vi "iWorx - Water Quality Lab.vi"() -> ()   [LabVIEW 2012]
uses:
  vi.lib/iWorx/iWorx Set Points.ctl
  <vilib>/Utility/miscctls.llb/LVRangeTypeDef.ctl
  <vilib>/DAQmx/create/channels.llb/DAQmx Create Channel (AI-Voltage-Basic).vi
  <vilib>/DAQmx/read.llb/DAQmx Read (Analog 1D Wfm NChan 1Samp).vi
panel:
  in  "Reset Scale":bool
  in  "Log Info Button":bool
  in  "Stop":bool
  in  "Reset Default Cal":bool
  in  "Set Points":T1={"SP1 Voltage"=0.2, "SP1 Value"=20.0, "SP2 Voltage"=2.0, "SP2 Value"=200.0} {"SP2 Value" format="%.1f"; "SP2 Voltage" format="%.2f V"; "SP1 Value" format="%.1f"; "SP1 Voltage" format="%.2f V"}
  out "Offset(b)":dbl=-1.1111111111111112
  out "Slope(m)":dbl=5.277777777777778
  in  "Sensor":u16(ring) items=["Dissolved Oxygen", "pH", "Conductivity", "Turbidity"]
  in  "Set Up":bool
  in  "Pause Button":bool
  in  "Snapshot":bool
  out "Processed Signal":dbl(knob) caption="Oxygen Content" scale=0.0..100.0 scale format="%#_6p"
  out "Waveform Chart":waveform(dbl)(graph)
  in  "Sample Timing":u16(ring)=200 items=["20Hz"=50, "5 Hz"=200, "2 Hz"=500, "1 Hz"=1000, ".5 Hz"=2000, ".2 Hz"=5000]
  in  "Clear Chart":bool
  in  "Open Log":bool
  in  "Rescale Y":bool
  out "Raw Signal":dbl(knob) scale=-5.0..5.0
  # "Water Quality Lab"
  # "Sensor Input (Ch 1)"
  # "(            ,            )"
  # "(            ,            )"
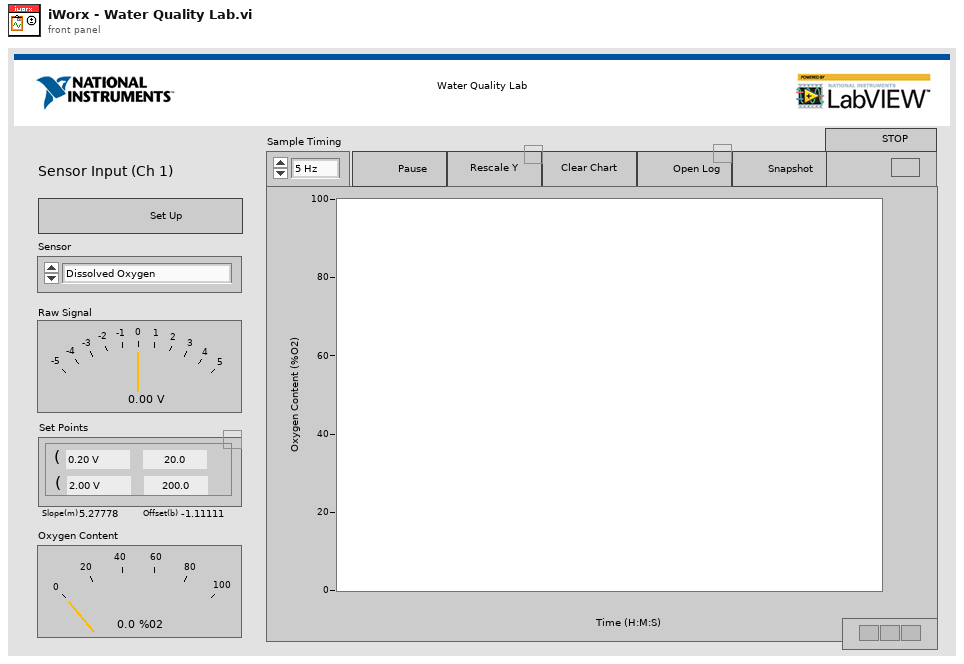
[diagram p1: front panel]
types:
  T1 = typedef "iWorx Set Points.ctl" = cluster{"SP1 Voltage":dbl, "SP1 Value":dbl, "SP2 Voltage":dbl, "SP2 Value":dbl}
  T2 = typedef "LVRangeTypeDef.ctl" = cluster{"Minimum":dbl, "Maximum":dbl, "Increment":dbl, "Minor Increment":dbl, "Start":dbl}
  T3 = cluster{"Name":string, "Format String":string, "Y Scale Name":string, "Scale.Range":T2, "Calibration Data":cluster{"SP1 Voltage":dbl, "SP2 Voltage":dbl, "SP1 Value":dbl, "SP2 Value":dbl}}[]
  T4 = cluster{"Name":string, "Format String":string, "Y Scale Name":string, "Scale.Range":T2, "Calibration Data":cluster{"SP1 Voltage":dbl, "SP2 Voltage":dbl, "SP1 Value":dbl, "SP2 Value":dbl}}
  T5 = cluster{"SP1 Voltage":dbl, "SP2 Voltage":dbl, "SP1 Value":dbl, "SP2 Value":dbl}
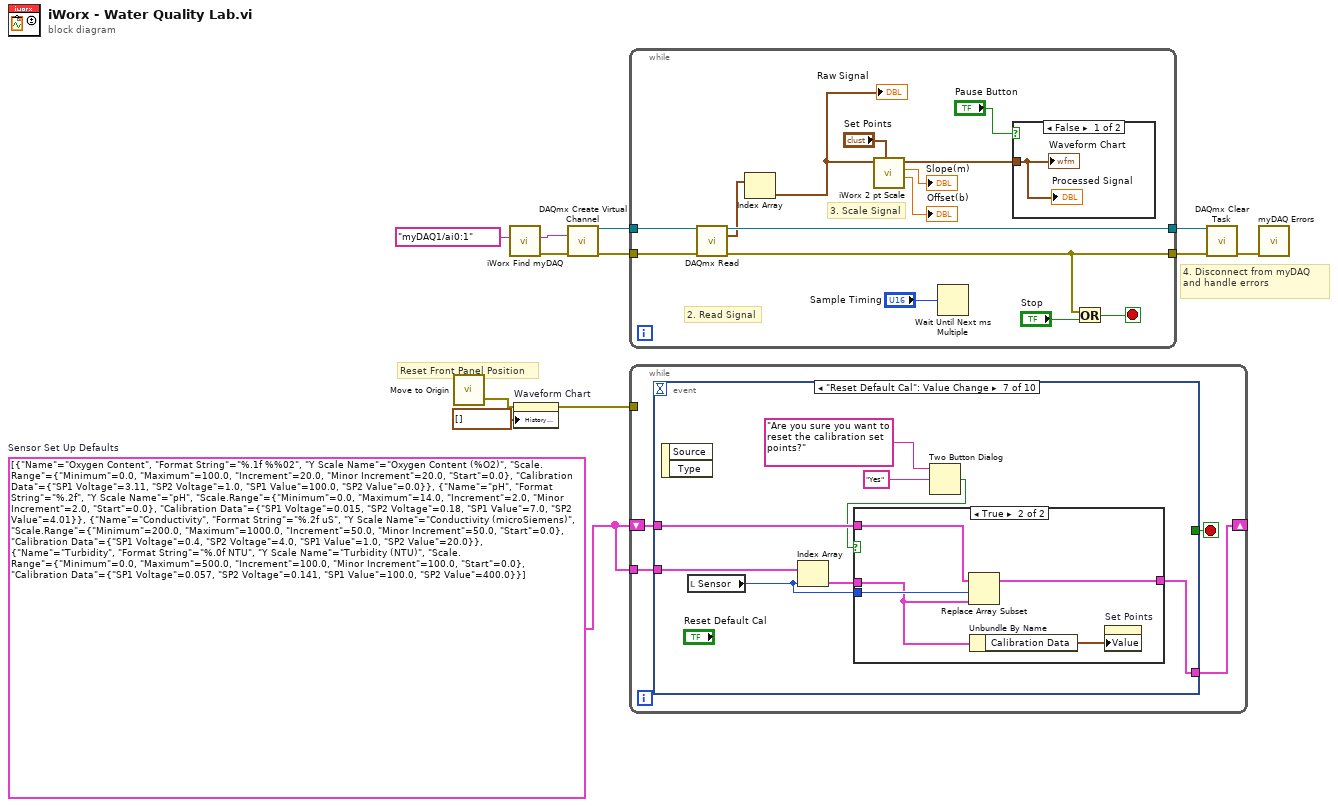
[diagram p0: block diagram]
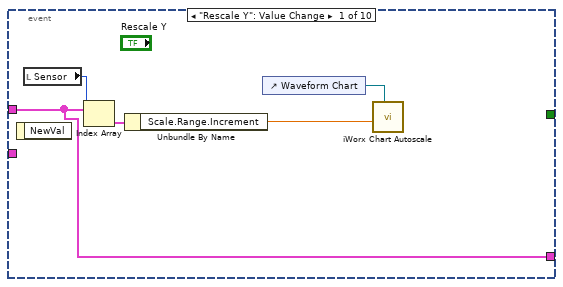
[diagram p2: hidden frame]
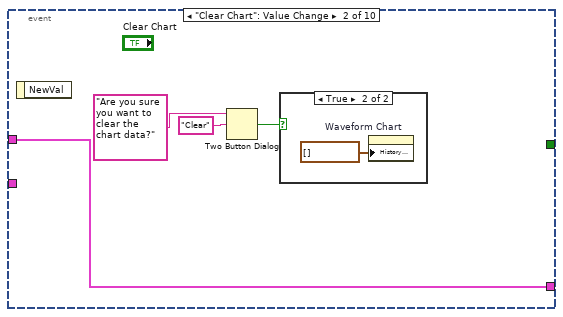
[diagram p3: hidden frame]
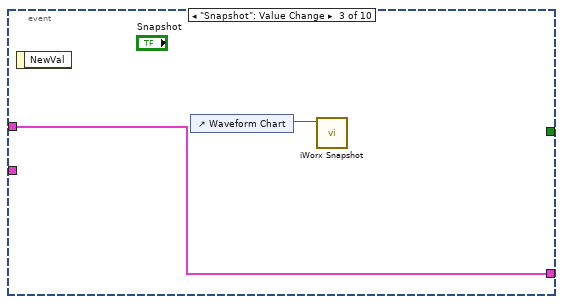
[diagram p5: hidden frame]
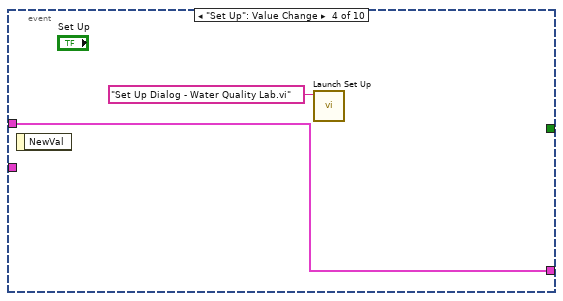
[diagram p6: hidden frame]
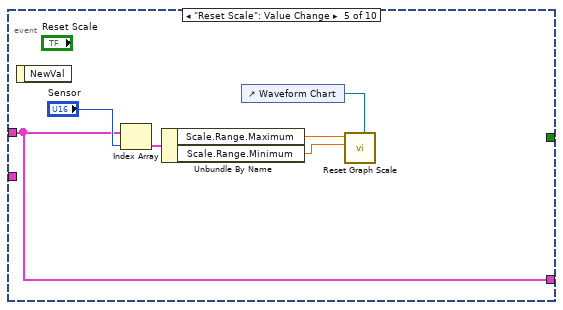
[diagram p7: hidden frame]
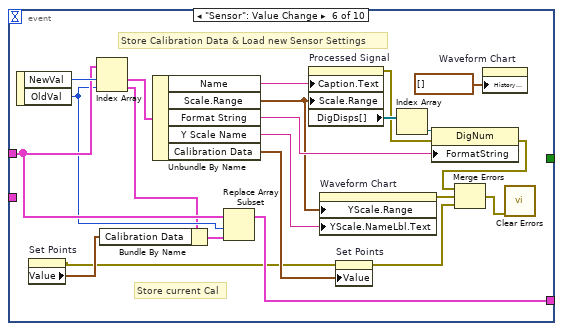
[diagram p8: hidden frame]
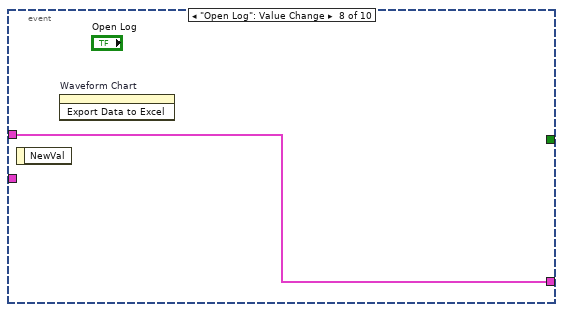
[diagram p10: hidden frame]
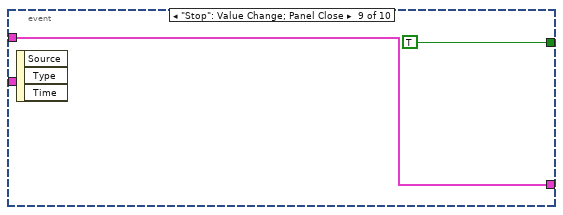
[diagram p11: hidden frame]
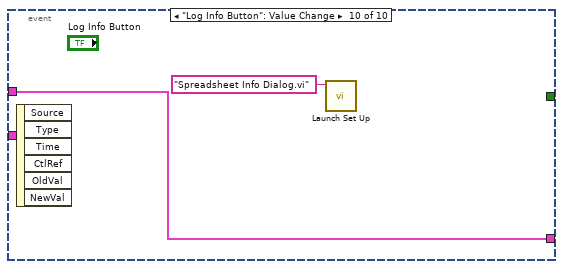
[diagram p12: hidden frame]
diagram:
  w1 = T3 [{"Name"="Oxygen Content", "Format String"="%.1f %%02", "Y Scale Name"="Oxygen Content (%O2)", "Scale.Range"={"Minimum"=0.0, "Maximum"=100.0, "Increment"=20.0, "Minor Increment"=20.0, "Start"=0.0}, "Calibration Data"={"SP1 Voltage"=3.11, "SP2 Voltage"=1.0, "SP1 Value"=100.0, "SP2 Value"=0.0}}, {"Name"="pH", "Format String"="%.2f", "Y Scale Name"="pH", "Scale.Range"={"Minimum"=0.0, "Maximum"=14.0, "Increment"=2.0, "Minor Increment"=2.0, "Start"=0.0}, "Calibration Data"={"SP1 Voltage"=0.015, "SP2 Voltage"=0.18, "SP1 Value"=7.0, "SP2 Value"=4.01}}, {"Name"="Conductivity", "Format String"="%.2f uS", "Y Scale Name"="Conductivity (microSiemens)", "Scale.Range"={"Minimum"=200.0, "Maximum"=1000.0, "Increment"=50.0, "Minor Increment"=50.0, "Start"=0.0}, "Calibration Data"={"SP1 Voltage"=0.4, "SP2 Voltage"=4.0, "SP1 Value"=1.0, "SP2 Value"=20.0}}, {"Name"="Turbidity", "Format String"="%.0f NTU", "Y Scale Name"="Turbidity (NTU)", "Scale.Range"={"Minimum"=0.0, "Maximum"=500.0, "Increment"=100.0, "Minor Increment"=100.0, "Start"=0.0}, "Calibration Data"={"SP1 Voltage"=0.057, "SP2 Voltage"=0.141, "SP1 Value"=100.0, "SP2 Value"=400.0}}]  # Sensor Set Up Defaults
  # "Reset Front Panel Position"
  # "4. Disconnect from myDAQ and handle errors"
  n1 = call "Move to Origin.vi"() -> ("Error Out"=w2:errorcluster)  [unwired: 3 in]
  n2 = call "iWorx Find myDAQ.vi"("Preferred myDAQ (myDAQ1)"=tag "myDAQ1/ai0:1" ("physical channels")) -> ("Error Out"=w5:errorcluster, "DAQmx Physical Channel"=w6:tag)  [unwired: 6 in, 3 out]
  n3 = property on="Waveform Chart" class="WFChart (strict)"(error in=w2, "History Data"=waveform(dbl)[] []) -> (error out=w8:errorcluster)  [unwired: 1 in, 1 out]
  n4 = call-poly <vilib>:"DAQmx Create Virtual Channel.vi"("physical channels"=w6, "error in"=w5) -> ("task out"=w10:refnum<k21>, "error out"=w9:errorcluster)  [unwired: 12 in]
  n5 = while {
    tunnel: w10 -> [w25]
    tunnel: [w24] -> w12
    tunnel: w9 -> [w23]
    tunnel: [w21] -> w11
    stop <- w22 stop-if-true
    # "3. Scale Signal"
    # "2. Read Signal"
    n6 = call-poly <vilib>:"DAQmx Read.vi"("task/channels in"=w25, "error in"=w23) -> ("task out"=w24:refnum<k21>, "data"=w19:waveform(dbl)[], "error out"=w21:errorcluster)  [unwired: 11 in]
    n7 = Index Array(array=w19) -> (element=w17:waveform(dbl))  [unwired: 1 in]
    "Raw Signal" <- w17
    n8 = call "iWorx 2 pt Scale.vi"("Set Points"="Set Points", "Raw Waveform"=w17) -> ("Offset"=→"Offset(b)":dbl, "Slope"=→"Slope(m)":dbl, "Scaled Value"=w18:waveform(dbl))  [unwired: 7 in]
    n9 = Wait Until Next ms Multiple(millisecond multiple="Sample Timing") -> ()  [unwired: 1 out]
    n10 = case shown="False" "Pause Button" {
      tunnel: w18 -> [w27 _]
      frame False {
        "Waveform Chart" <- w27
        "Processed Signal" <- w27
      }
      frame True {
      }
    }
    n11 = Or(x=w21, y="Stop") -> (x .or. y?=w22:bool)
  }
  n12 = while {
    tunnel: w8 -> [_]
    shift-right: [w29] -> _
    shift-left: w1 -> [w30]
    tunnel: w1 -> [w28]
    stop <- w31 stop-if-true
    n13 = event shown="[6] \"Reset Default Cal\": Value Change" {
      selector: _ -> [_ _ _ _ _ _ _ _ _ _]
      dyn-events: _ -> [_ _ _ _ _ _ _ _ _ _]
      timeout: _ -> [_ _ _ _ _ _ _ _ _ _]
      tunnel: [_ _ _ _ _ _ _ _ TRUE _] -> w31
      tunnel: w30 -> [w32 w37 w42 w44 w46 w66 w78 w88 w89 w91]
      tunnel: [w32 w37 w42 w44 w46 w63 w75 w88 w89 w91] -> w29
      tunnel: w28 -> [_ _ _ _ _ _ w79 _ _ _]
      event "Rescale Y": Value Change {
        n14 = event-data() -> ()  [unwired: 1 in, 1 out]
        n15 = local read "Sensor"() -> (w34:u16)
        n16 = Index Array(array=w32, index=w34) -> (element=w35:T4)
        n17 = Unbundle By Name(w35) -> ("Scale.Range.Increment"=w33:dbl)
        n18 = control-ref of="Waveform Chart"() -> (w36:refnum<vi>)
        n19 = call "iWorx Chart Autoscale.vi"("Selection Chart"=w36, "Rounding Multiple (10)"=w33) -> ()  [unwired: 7 in, 3 out]
      }
      event "Clear Chart": Value Change {
        n20 = event-data() -> ()  [unwired: 1 in, 1 out]
        n21 = Two Button Dialog(message="Are you sure you want to clear the chart data?", 2:"Clear" ("T button name (\"OK\")")) -> (T button?=w39:bool)  [unwired: 1 in]
        n22 = case shown="True" w39 {
          frame False {
          }
          frame True {
            n23 = property on="Waveform Chart" class="WFChart (strict)"("History Data"=waveform(dbl)[] []) -> ()  [unwired: 2 in, 2 out]
          }
        }
      }
      event "Snapshot": Value Change {
        n24 = event-data() -> ()  [unwired: 1 in, 1 out]
        n25 = control-ref of="Waveform Chart"() -> (w43:refnum<vi>)
        n26 = call "iWorx Snapshot.vi"("WaveformChart in"=w43) -> ()  [unwired: 10 in, 1 out]
      }
      event "Set Up": Value Change {
        n27 = event-data() -> ()  [unwired: 1 in, 1 out]
        n28 = call "Launch Set Up.vi"("name or relative path"="Set Up Dialog - Water Quality Lab.vi") -> ()  [unwired: 9 in, 2 out]
      }
      event "Reset Scale": Value Change {
        n29 = event-data() -> ()  [unwired: 1 in, 1 out]
        n30 = Index Array(array=w46, index="Sensor") -> (element=w49:T4)
        n31 = Unbundle By Name(w49) -> ("Scale.Range.Maximum"=w48:dbl, "Scale.Range.Minimum"=w47:dbl)
        n32 = control-ref of="Waveform Chart"() -> (w51:refnum<vi>)
        n33 = call "Reset Graph Scale.vi"("WaveformChart in"=w51, "Minimum (0)"=w47, "Maximum (100)"=w48) -> ()  [unwired: 8 in, 1 out]
      }
      event "Sensor": Value Change {
        # "Store current Cal"
        # "Store Calibration Data & Load new Sensor Settings"
        n34 = event-data() -> ("NewVal"=w67:u16, "OldVal"=w64:u16)  [unwired: 1 in]
        n35 = property on="Set Points" class="Clust (strict)"() -> (error out=w53:errorcluster, "Value"=w55:T1)  [unwired: 2 in, 1 out]
        n36 = Index Array(array=w66, index #1=w67, index #2=w64) -> (element #1=w65:T4, element #2=w60:T4)
        n37 = Bundle By Name(cluster=w60, "Calibration Data"=w55) -> (w62:T4)
        n38 = Unbundle By Name(w65) -> ("Name"=w71:string, "Scale.Range"=w69:T2, "Format String"=w70:string, "Y Scale Name"=w68:string, "Calibration Data"=w54:T5)
        n39 = Replace Array Subset(array=w66, new element=w62, index=w64) -> (w63:T3)
        n40 = property on="Processed Signal" class="Knob (strict)"("Caption.Text"=w71, "Scale.Range"=w69) -> (error out=w59:errorcluster, "DigDisps[]"=w72:refnum<vi>[])  [unwired: 2 in, 1 out]
        n41 = property on="Waveform Chart" class="WFChart (strict)"("YScale.Range"=w69, "YScale.NameLbl.Text"=w68) -> (error out=w57:errorcluster)  [unwired: 2 in, 1 out]
        n42 = property on="Set Points" class="Clust (strict)"(error in=w53, "Value"=w54) -> (error out=w52:errorcluster)  [unwired: 1 in, 1 out]
        n43 = Index Array(array=w72) -> (element=w73:refnum<vi>)  [unwired: 1 in]
        n44 = property class="DigNum"(reference=w73, error in=w59, "FormatString"=w70) -> (error out=w58:errorcluster)  [unwired: 1 out]
        n45 = Merge Errors(w58, w57, w52) -> (w56:errorcluster)
        n46 = property on="Waveform Chart" class="WFChart (strict)"("History Data"=waveform(dbl)[] []) -> ()  [unwired: 2 in, 2 out]
        n47 = call <vilib>:"Clear Errors.vi"("error in (no error)"=w56) -> ()  [unwired: 6 in, 1 out]
      }
      event "Reset Default Cal": Value Change {
        n48 = event-data() -> ()  [unwired: 1 in, 2 out]
        n49 = local read "Sensor"() -> (w77:u16)
        n50 = Index Array(array=w79, index=w77) -> (element=w76:T4)
        n51 = Two Button Dialog(message="Are you sure you want to reset the calibration set points?", 2:"Yes" ("T button name (\"OK\")")) -> (T button?=w74:bool)  [unwired: 1 in]
        n52 = case shown="True" w74 {
          tunnel: w78 -> [w82 w87]
          tunnel: w77 -> [_ w86]
          tunnel: w76 -> [_ w85]
          tunnel: [w82 w83] -> w75
          frame False {
          }
          frame True {
            n53 = Replace Array Subset(array=w87, new element=w85, index=w86) -> (w83:T3)
            n54 = Unbundle By Name(w85) -> ("Calibration Data"=w84:T5)
            n55 = property on="Set Points" class="Clust (strict)"("Value"=w84) -> ()  [unwired: 2 in, 2 out]
          }
        }
      }
      event "Open Log": Value Change {
        n56 = event-data() -> ()  [unwired: 1 in, 1 out]
        n57 = invoke on="Waveform Chart" class="WFChart (strict)" method="Export Data to Excel"() -> ()  [unwired: 3 in, 3 out]
      }
      event "Stop": Value Change; Panel Close {
        n58 = event-data() -> ()  [unwired: 1 in, 3 out]
      }
      event "Log Info Button": Value Change {
        n59 = event-data() -> ()  [unwired: 1 in, 6 out]
        n60 = call "Launch Set Up.vi"("name or relative path"="Spreadsheet Info Dialog.vi") -> ()  [unwired: 9 in, 2 out]
      }
    }
  }
  n61 = call <vilib>:"DAQmx Clear Task.vi"("task in"=w12, "error in"=w11) -> ("error out"=w3:errorcluster)  [unwired: 13 in]
  n62 = call "myDAQ Errors.vi"("error in (no error)"=w3) -> ()  [unwired: 10 in, 1 out]
